vi "PH_Switch.get i attribute.vi"(0 "i ref in":refnum<vi>, 5 "error in (no error)":errorcluster) -> (14 "i ref out":refnum<vi>, 16 "i attribute":T1={"GUI Refs"={"true"=refnum, "false"=refnum, "Switch_state"=refnum, "GUI-Knob"=refnum, "Delete"=refnum, "Function Textfield"=refnum}, "Status true"=0, "Status false"=0, "Status Switch State"=0, "remote controlled"=FALSE, "Tagname"={"Switch"="N/A", "True"="N/A", "False"="N/A"}, "Beckhoff Instance"="N/A", "Caption"={"True"="", "False"=""}, "Default State"="N/A"} {"Status Switch State" items=["no info", "off/false/out", "on/true/in", "Failure", "Alarm", "Status 1", "Status 2", "Status 3"]; "Status false" items=["no info", "off/false/out", "on/true/in", "Failure", "Alarm", "Status 1", "Status 2", "Status 3"]; "Status true" items=["no info", "off/false/out", "on/true/in", "Failure", "Alarm", "Status 1", "Status 2", "Status 3"]}, 19 "error out":errorcluster)   [LabVIEW 2014, in "PH_Switch.lvlib"]
doc: "Gets the i attribute data of an object.\n\nLicense Agreement for this software:\n\nCopyright (C)\nGesellschaft für Schwerionenforschung, GSI\nPlanckstr. 1\n64291 Darmstadt\nGermany\n\nContact: D.Beck@gsi.de \n\nThis program is free software; you can redistribute it and/or modify it under the terms of the GNU General Public License as published by the Free Software Foundation; either version 2 of the license, or (at your option) any later version.\n\nThis program is distributed in the hope that it will be useful, but WITHOUT ANY WARRANTY; without even the implied warranty of MERCHANTABILITY or FITNESS FOR A PARTICULAR PURPOSE. See the GNU General License for more details (http://www.gnu.org).\n\nGesellschaft für Schwerionenforschung, GSI\nPlanckstr. 1, 64291 Darmstadt, Germany\nFor all questions and ideas contact: M.Richter@gsi.de, H.Brand@gsi.de or D.Beck@gsi.de.\nLast update: 17-JUN-2004"
uses:
  PH_Switch.lvlib
  PH_Switch.i attribute.ctl
  PH_Switch.GUI Refs.ctl
  PH_Basics/PH_StatusHandler/PH_StatusHandler.Status.ctl
  PH_Basics/PH_StatusHandler/PH_StatusHandler.lvlib
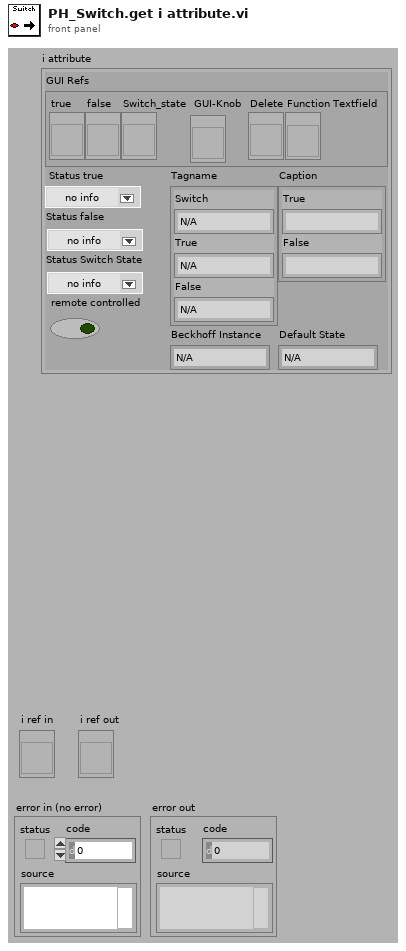
[diagram p1: front panel]
types:
  T1 = typedef "PH_Switch.lvlib/PH_Switch.i attribute.ctl" = cluster{"GUI Refs":T2, "Status true":T3, "Status false":T3, "Status Switch State":T3, "remote controlled":bool, "Tagname":cluster{"Switch":string, "True":string, "False":string}, "Beckhoff Instance":string, "Caption":cluster{"True":string, "False":string}, "Default State":string}
  T2 = typedef "PH_Switch.lvlib/PH_Switch.GUI Refs.ctl" = cluster{"true":refnum<vi>, "false":refnum<vi>, "Switch_state":refnum<vi>, "GUI-Knob":refnum<vi>, "Delete":refnum<vi>, "Function Textfield":refnum<vi>}
  T3 = typedef "PH_StatusHandler.lvlib/PH_StatusHandler.Status.ctl" = i16
  T4 = enum16{"SetAttribute", "GetAttribute", "CreateAttribute", "DestroyAttribute", "DestroyAllAtributes"}
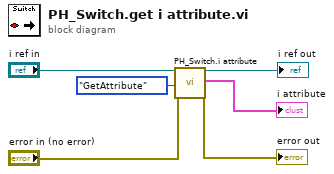
[diagram p0: block diagram]
diagram:
  n1 = call "PH_Switch.i attribute.vi"("VI Refnum"="i ref in", "Action"=T4."GetAttribute", "error in (no error)"="error in (no error)") -> ("VI Refnum out"=→"i ref out":refnum<vi>, "CLASS.i attribute out"=→"i attribute":T1, "error out"=→"error out":errorcluster)  [unwired: 14 in]
